vi "test_camera_MAKO.vi"(0 "Boolean 2":bool, 1 "Exposure_set":dbl, 2 "Slide 2":dbl(slide) scale=35.0..1000.0, 3 "Value_Set (ms)":bool, 4 "Bar_Set (ms)":bool, 6 "STOP":bool, 8 "PAUSE":bool, 10 "SAVE PHOTO":bool, 12 "Path":path, 14 "Boolean":bool, 15 "Gain_Set":dbl, 16 "Slide 3":dbl(slide) scale=0.0..30.0, 17 "Bar_Set (dB)":bool, 18 "Value_Set (dB)":bool) -> (5 "gain":dbl, 13 "new picture":picture, 19 "exposure":dbl)   [LabVIEW 2026]
uses:
  <vilib>/picture/picture.llb/Draw True-Color Pixmap.vi
  <userlib>/MakoWrapper/MakoWrapper.lvlib
panel:
  in  "Tab Control 2":enum32{"Image", "Exposure", "Gain"}(tab)
  out "Frame Rate (Hz)":i8
  in  "Duration":dbl
  out "Boolean 3":bool
  out "Frame Flicker":bool
  in  "Start_Video":bool
  in  "Duratin_Video":bool
  out "Auto_Expose":bool
  out "Auto_Gain":bool
  in  "Tab Control":T1(tab)
  out "error_start":errorcluster
  out "start_return":i32
  in  "cameraId":string="DEV_000F315E8832"
  out "error_open":errorcluster
  out "open_return":i32
  out "setup_return":i32
  out "error_setup":errorcluster
  out "error out":errorcluster
  out "error_sizing":errorcluster
  in  "timeoutMs":u32=2000
  in  "bufferSize":u32=4986432
  out "size_return":i32
  out "width":i32
  out "height":i32
  out "outBuffer":u8[](array[numeric])
  out "error_cam_close":errorcluster
  out "cam_close_return":i32
  out "error_shutdown":errorcluster
  out "shutdown_return":i32
  out "error_exposure":errorcluster
  out "exposure_return":i32
  out "error_gain":errorcluster
  out "gain_return":i32
  # "DEV_000F315E8832"
  # "4986432"
  # "2000"
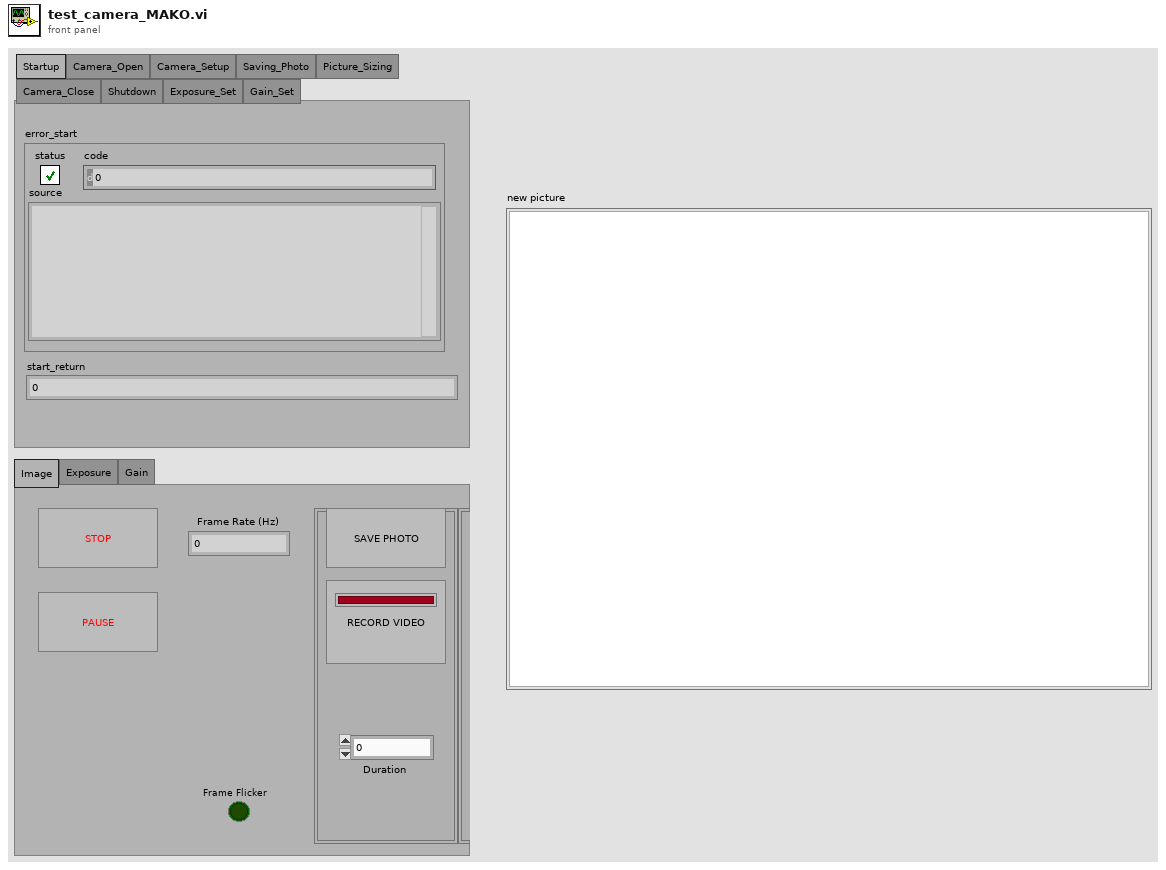
[diagram p1: front panel]
types:
  T1 = enum32{"Startup", "Camera_Open", "Camera_Setup", "Saving_Photo", "Picture_Sizing", "Camera_Close", "Shutdown", "Exposure_Set", "Gain_Set"}
  T2 = typedef "imagedata.ctl" = cluster{"image type":i32, "image depth":i32, "image":u8[], "mask":u8[], "colors":u32[], "Rectangle":cluster{"left":i16, "top":i16, "right":i16, "bottom":i16}}
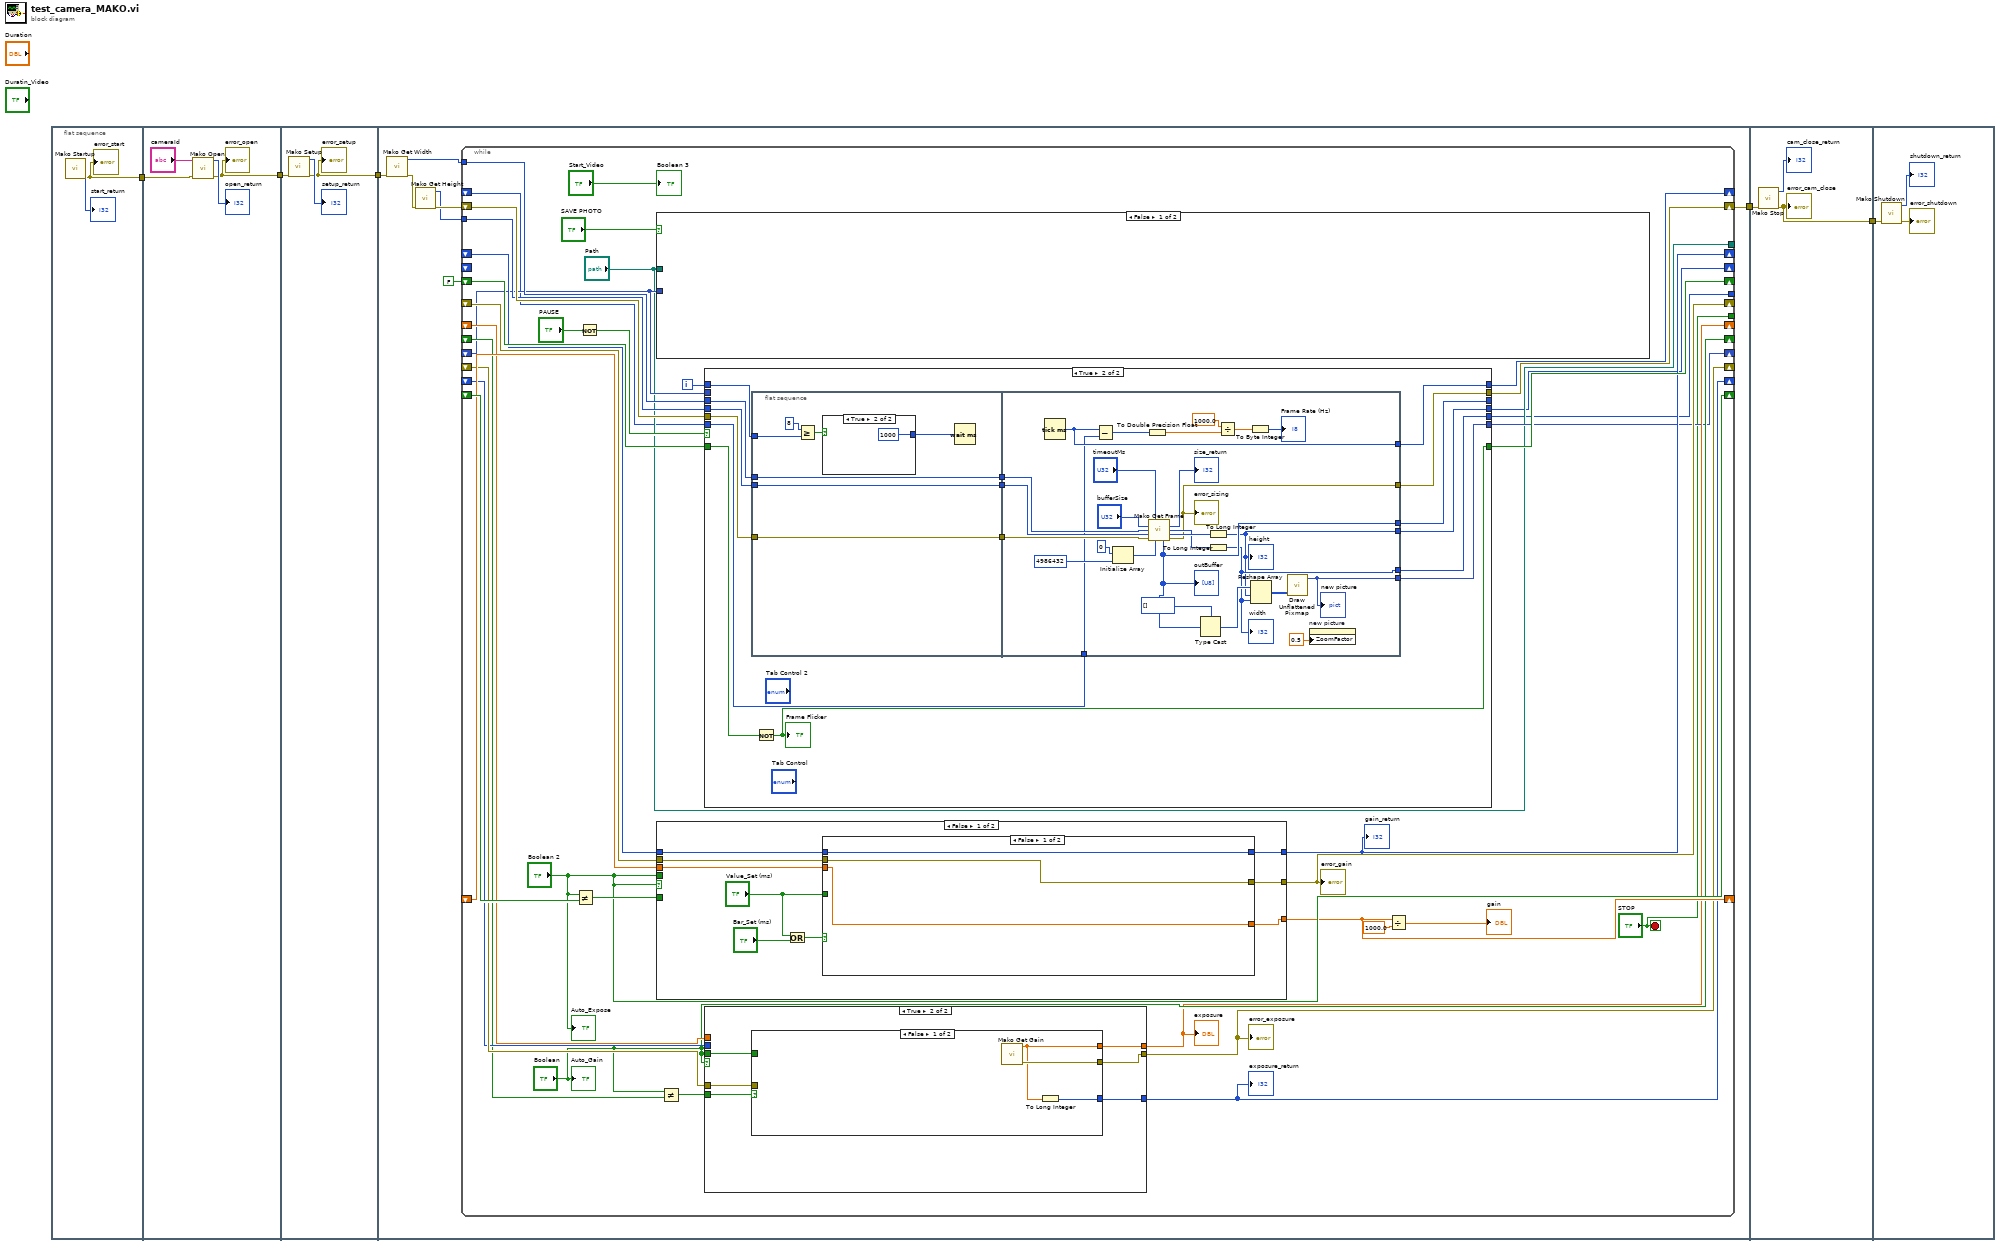
[diagram p0: block diagram]
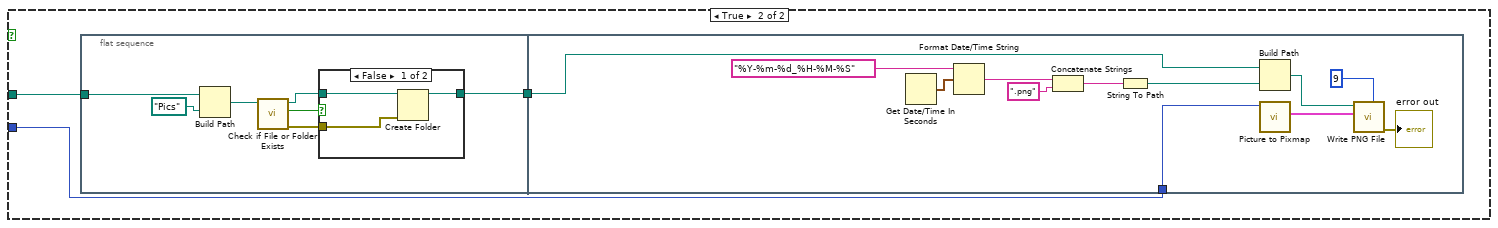
[diagram p2: hidden frame]
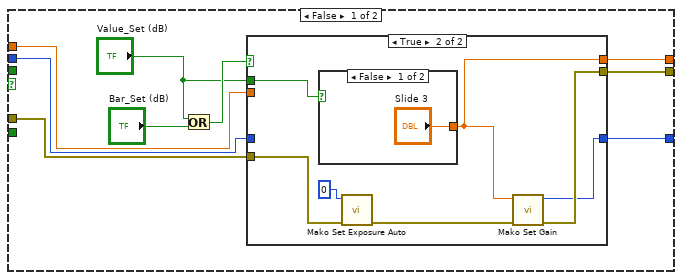
[diagram p4: hidden frame]
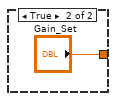
[diagram p6: hidden frame]
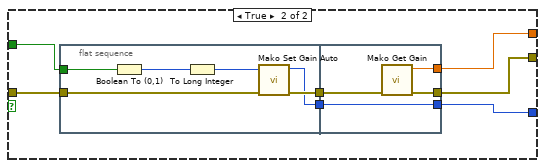
[diagram p7: hidden frame]
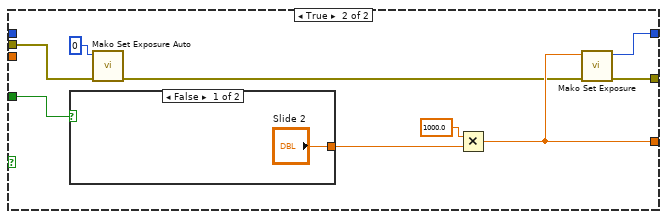
[diagram p8: hidden frame]
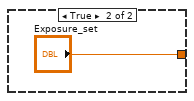
[diagram p9: hidden frame]
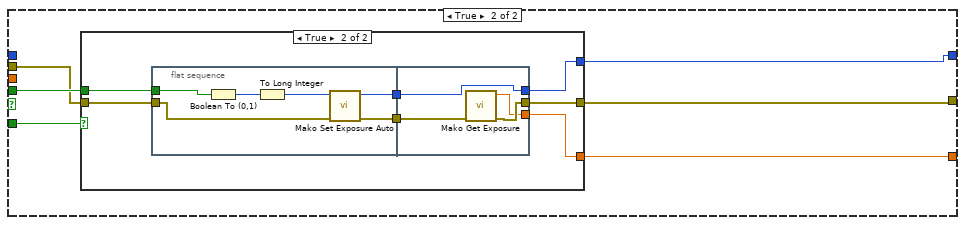
[diagram p10: hidden frame]
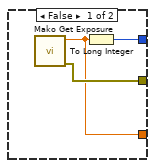
[diagram p11: hidden frame]
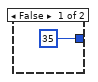
[diagram p13: hidden frame]
diagram:
  n1 = flat-sequence {
    tunnel: [w6] -> w5
    tunnel: w5 -> [w8]
    tunnel: [w9] -> w4
    tunnel: w4 -> [w14]
    tunnel: [w12] -> w3
    tunnel: w3 -> [w21]
    tunnel: [w16] -> w2
    tunnel: w2 -> [w241]
    tunnel: [w239] -> w1
    tunnel: w1 -> [w244]
    frame #0 {
      n2 = call <userlib>:"Mako Startup.vi"() -> ("error out"=w6:errorcluster, "function return"=→"start_return":i32)  [unwired: 10 in]
      "error_start" <- w6
    }
    frame #1 {
      n3 = call <userlib>:"Mako Open.vi"("error in (no error)"=w8, "cameraId"="cameraId") -> ("error out"=w9:errorcluster, "function return"=→"open_return":i32)  [unwired: 8 in]
      "error_open" <- w9
    }
    frame #2 {
      n4 = call <userlib>:"Mako Setup.vi"("error in (no error)"=w14) -> ("error out"=w12:errorcluster, "function return"=→"setup_return":i32)  [unwired: 9 in]
      "error_setup" <- w12
    }
    frame #3 {
      n5 = call <userlib>:"Mako Get Width.vi"("error in (no error)"=w21) -> ("error out"=w20:errorcluster, "function return"=w18:u32)  [unwired: 9 in]
      n6 = call <userlib>:"Mako Get Height.vi"("error in (no error)"=w20) -> ("error out"=w19:errorcluster, "function return"=w17:u32)  [unwired: 9 in]
      n7 = while {
        tunnel: w18 -> [w59]
        tunnel: w17 -> [w58]
        shift-right: [w57] -> w16
        shift-left: w19 -> [w60]
        shift-right: [w52] -> _
        shift-left: FALSE -> [w53]
        shift-right: ["Boolean 2"] -> _
        shift-left: _ -> [w51]
        shift-right: [w48] -> _
        shift-left: _ -> [w47]
        shift-right: [w46] -> _
        shift-left: _ -> [w45]
        shift-right: [w44] -> _
        shift-left: _ -> [w43]
        shift-right: ["Boolean"] -> _
        shift-left: _ -> [w38]
        shift-right: [w36] -> _
        shift-left: _ -> [w40]
        shift-right: [w35] -> _
        shift-left: _ -> [w41]
        shift-right: [w32] -> _
        shift-left: _ -> [w42]
        shift-right: [w30] -> _
        shift-left: _ -> [w29]
        tunnel: ["Path"] -> _
        tunnel: [w26] -> _
        tunnel: ["STOP"] -> _
        shift-right: [w23] -> _
        shift-left: _ -> [w22]
        shift-right: [w25] -> _
        shift-left: _ -> [_]
        i -> [w56]
        stop <- "STOP" stop-if-true
        n8 = Not Equal?(x="Boolean 2", y=w51) -> (x != y?=w50:bool)
        n9 = Not(x="PAUSE") -> (.not. x?=w54:bool)
        n10 = case shown="False" "SAVE PHOTO" {
          tunnel: w29 -> [_ w62]
          tunnel: "Path" -> [_ w61]
          frame False {
          }
          frame True {
            n11 = flat-sequence {
              tunnel: w61 -> [w69]
              tunnel: [w65] -> w63
              tunnel: w63 -> [w84]
              tunnel: w62 -> [w76]
              frame #0 {
                n12 = Build Path(base path=w69, name or relative path=path "Pics") -> (appended path=w64:path)
                n13 = call <vilib>:"Check if File or Folder Exists.vi"("path"=w64) -> ("error out"=w66:errorcluster, "file or folder exists?"=w68:bool, "dup path"=w67:path)  [unwired: 8 in]
                n14 = case shown="False" w68 {
                  tunnel: w67 -> [w73 w74]
                  tunnel: w66 -> [w72 _]
                  tunnel: [w71 w74] -> w65
                  frame False {
                    n15 = Create Folder(path (use dialog)=w73, error in=w72) -> (created path=w71:path)  [unwired: 1 in, 2 out]
                  }
                  frame True {
                  }
                }
              }
              frame #1 {
                n16 = Get Date/Time In Seconds() -> (seconds since 1Jan1904=w86:timestamp)
                n17 = Format Date/Time String(time format string (%c)="%Y-%m-%d_%H-%M-%S", seconds (now)=w86) -> (date/time string=w81:string)  [unwired: 1 in]
                n18 = Concatenate Strings(w81, ".png" ("string")) -> (w82:string)
                n19 = String To Path(string=w82) -> (path=w78:path)
                n20 = Build Path(base path=w84, name or relative path=w78) -> (appended path=w79:path)
                n21 = call <vilib>:"Picture to Pixmap.vi"("picture"=w76) -> ("image data"=w83:T2)  [unwired: 9 in, 1 out]
                n22 = call <vilib>:"Write PNG File.vi"("compression (default)"=9, "image data"=w83, "path to PNG file"=w79) -> ("error out"=→"error out":errorcluster)  [unwired: 7 in, 1 out]
              }
            }
          }
        }
        n23 = case shown="False" "Boolean 2" {
          tunnel: [w139 w158] -> w44
          tunnel: w50 -> [_ w162]
          tunnel: "Boolean 2" -> [_ w161]
          tunnel: [w138 w160] -> w46
          tunnel: [w137 w159] -> w48
          tunnel: w47 -> [w136 _]
          tunnel: w45 -> [w135 w157]
          tunnel: w43 -> [w134 _]
          frame False {
            n24 = Or(x="Value_Set (ms)", y="Bar_Set (ms)") -> (x .or. y?=w142:bool)
            n25 = case shown="False" w142 {
              tunnel: [w143 w150] -> w139
              tunnel: "Value_Set (ms)" -> [_ w154]
              tunnel: [w144 w153] -> w138
              tunnel: [w145 w152] -> w137
              tunnel: w136 -> [w145 _]
              tunnel: w135 -> [w144 w148]
              tunnel: w134 -> [w143 _]
              frame False {
              }
              frame True {
                n26 = case shown="False" w154 {
                  tunnel: ["Slide 2" "Exposure_set"] -> w151
                  frame False {
                  }
                  frame True {
                  }
                }
                n27 = call <userlib>:"Mako Set Exposure Auto.vi"("error in (no error)"=w148, "autoOn"=0) -> ("error out"=w147:errorcluster)  [unwired: 8 in, 1 out]
                n28 = Multiply(x=1000.0, y=w151) -> (x*y=w150:dbl)
                n29 = call <userlib>:"Mako Set Exposure.vi"("error in (no error)"=w147, "exposureUs"=w150) -> ("error out"=w153:errorcluster, "function return"=w152:i32)  [unwired: 8 in]
              }
            }
          }
          frame True {
            n30 = case shown="True" w162 {
              tunnel: w161 -> [_ w172]
              tunnel: [w165 w171] -> w160
              tunnel: [w164 w170] -> w159
              tunnel: [w163 w167] -> w158
              tunnel: w157 -> [_ w166]
              frame False {
                n31 = call <userlib>:"Mako Get Exposure.vi"() -> ("error out"=w165:errorcluster, "function return"=w163:dbl)  [unwired: 10 in]
                n32 = To Long Integer(number=w163) -> (32bit integer=w164:i32)
              }
              frame True {
                n33 = flat-sequence {
                  tunnel: w172 -> [w178]
                  tunnel: [w175] -> w169
                  tunnel: [w174] -> w168
                  tunnel: w166 -> [w173]
                  tunnel: [w182] -> w170
                  tunnel: [w180] -> w171
                  tunnel: w169 -> [w181]
                  tunnel: w168 -> [w182]
                  tunnel: [w179] -> w167
                  frame #0 {
                    n34 = Boolean To (0,1)(Boolean=w178) -> (0, 1=w177:i16)
                    n35 = To Long Integer(number=w177) -> (32bit integer=w176:i32)
                    n36 = call <userlib>:"Mako Set Exposure Auto.vi"("error in (no error)"=w173, "autoOn"=w176) -> ("error out"=w175:errorcluster, "function return"=w174:i32)  [unwired: 8 in]
                  }
                  frame #1 {
                    n37 = call <userlib>:"Mako Get Exposure.vi"("error in (no error)"=w181) -> ("error out"=w180:errorcluster, "function return"=w179:dbl)  [unwired: 9 in]
                  }
                }
              }
            }
          }
        }
        "error_gain" <- w46
        "gain_return" <- w48
        n38 = Not Equal?(x="Boolean", y=w38) -> (x != y?=w39:bool)
        n39 = case shown="True" w54 {
          tunnel: w60 -> [w186 w202]
          tunnel: w59 -> [_ w197]
          tunnel: w58 -> [_ w201]
          tunnel: [w186 w200] -> w57
          tunnel: w56 -> [_ w193]
          tunnel: w53 -> [w185 w199]
          tunnel: [w185 w198] -> w52
          tunnel: [w184 w192] -> w30
          tunnel: w29 -> [w184 _]
          tunnel: [_ w191] -> _
          tunnel: [_ w190] -> w26
          tunnel: [_ w189] -> w25
          tunnel: [w183 w188] -> w23
          tunnel: w22 -> [w183 w187]
          frame False {
          }
          frame True {
            n40 = flat-sequence {
              tunnel: w197 -> [w207]
              tunnel: w201 -> [w208]
              tunnel: w202 -> [w209]
              tunnel: [w209] -> w196
              tunnel: [w208] -> w195
              tunnel: [w207] -> w194
              tunnel: w193 -> [w203]
              tunnel: w196 -> [w238]
              tunnel: w195 -> [w226]
              tunnel: w194 -> [w225]
              tunnel: [w231] -> w200
              tunnel: [w223] -> w192
              tunnel: [w222] -> w191
              tunnel: [w221] -> w190
              tunnel: [w220] -> w189
              tunnel: [w218] -> w188
              tunnel: w187 -> [w217]
              frame #0 {
                n41 = Greater Or Equal?(x=8, y=w203) -> (x >= y?=w205:bool)
                n42 = case shown="True" w205 {
                  tunnel: [u32 35 ("milliseconds to wait") u32 1000 ("milliseconds to wait")] -> w204
                  frame False {
                  }
                  frame True {
                  }
                }
                n43 = Wait (ms)(milliseconds to wait=w204) -> ()  [unwired: 1 out]
              }
              frame #1 {
                n44 = Tick Count (ms)() -> (millisecond timer value=w218:u32)
                n45 = Subtract(x=w218, y=w217) -> (x-y=w219:u32)
                n46 = Initialize Array(u8 0 ("element"), 4986432 ("dimension size")) -> (w228:u8[])
                n47 = To Double Precision Float(number=w219) -> (double precision float=w214:dbl)
                n48 = call <userlib>:"Mako Get Frame.vi"("timeoutMs"="timeoutMs", "bufferSize"="bufferSize", "outWidth"=w225, "outHeight"=w226, "error in (no error)"=w238, "outBuffer"=w228) -> ("function return"=→"size_return":i32, "outWidth out"=w232:u32, "outHeight out"=w233:u32, "outBuffer 2"=w222:u8[], "error out"=w231:errorcluster)  [unwired: 5 in]
                "error_sizing" <- w231
                "outBuffer" <- w222
                n49 = Type Cast(type=u32[] [] ("data (RGB format)"), x=w222) -> (*(type *) &x=w235:u32[])
                n50 = To Long Integer(number=w233) -> (32bit integer=w220:i32)
                "height" <- w220
                n51 = To Long Integer(number=w232) -> (32bit integer=w221:i32)
                "width" <- w221
                n52 = Divide(x=1000.0, y=w214) -> (x/y=w216:dbl)
                n53 = To Byte Integer(number=w216) -> (8bit integer=→"Frame Rate (Hz)":i8)
                n54 = Reshape Array(w235, w220, w221) -> (w224:u32[][])
                n55 = call-poly <vilib>:"Draw Unflattened Pixmap.vi"("data (RGB format)"=w224) -> ("new picture"=w223:picture)  [unwired: 8 in]
                "new picture" <- w223
                n56 = property on="new picture" class="Pict"("ZoomFactor"=sgl 0.5 ("Zoom Factor")) -> ()  [unwired: 2 in, 2 out]
              }
            }
            n57 = Not(x=w199) -> (.not. x?=w198:bool)
            "Frame Flicker" <- w198
          }
        }
        n58 = case shown="True" "Boolean" {
          tunnel: [w94 w109] -> w32
          tunnel: w39 -> [_ w113]
          tunnel: "Boolean" -> [_ w112]
          tunnel: [w93 w111] -> w35
          tunnel: [w92 w110] -> w36
          tunnel: w40 -> [w91 _]
          tunnel: w41 -> [w90 w108]
          tunnel: w42 -> [w89 _]
          frame False {
            n59 = Or(x="Value_Set (dB)", y="Bar_Set (dB)") -> (x .or. y?=w95:bool)
            n60 = case shown="True" w95 {
              tunnel: [w96 w102] -> w94
              tunnel: "Value_Set (dB)" -> [_ w105]
              tunnel: [w97 w104] -> w93
              tunnel: [w98 w103] -> w92
              tunnel: w91 -> [w98 _]
              tunnel: w90 -> [w97 w100]
              tunnel: w89 -> [w96 _]
              frame False {
              }
              frame True {
                n61 = case shown="False" w105 {
                  tunnel: ["Slide 3" "Gain_Set"] -> w102
                  frame False {
                  }
                  frame True {
                  }
                }
                n62 = call <userlib>:"Mako Set Exposure Auto.vi"("error in (no error)"=w100, "autoOn"=0) -> ("error out"=w99:errorcluster)  [unwired: 8 in, 1 out]
                n63 = call <userlib>:"Mako Set Gain.vi"("error in (no error)"=w99, "gain"=w102) -> ("error out"=w104:errorcluster, "function return"=w103:i32)  [unwired: 8 in]
              }
            }
          }
          frame True {
            n64 = case shown="False" w113 {
              tunnel: w112 -> [_ w123]
              tunnel: [w116 w122] -> w111
              tunnel: [w115 w121] -> w110
              tunnel: [w114 w118] -> w109
              tunnel: w108 -> [_ w117]
              frame False {
                n65 = call <userlib>:"Mako Get Gain.vi"() -> ("error out"=w116:errorcluster, "function return"=w114:dbl)  [unwired: 10 in]
                n66 = To Long Integer(number=w114) -> (32bit integer=w115:i32)
              }
              frame True {
                n67 = flat-sequence {
                  tunnel: w123 -> [w129]
                  tunnel: [w126] -> w120
                  tunnel: [w125] -> w119
                  tunnel: w117 -> [w124]
                  tunnel: [w133] -> w121
                  tunnel: [w131] -> w122
                  tunnel: w120 -> [w132]
                  tunnel: w119 -> [w133]
                  tunnel: [w130] -> w118
                  frame #0 {
                    n68 = Boolean To (0,1)(Boolean=w129) -> (0, 1=w128:i16)
                    n69 = To Long Integer(number=w128) -> (32bit integer=w127:i32)
                    n70 = call <userlib>:"Mako Set Gain Auto.vi"("error in (no error)"=w124, "autoOn"=w127) -> ("error out"=w126:errorcluster, "function return"=w125:i32)  [unwired: 8 in]
                  }
                  frame #1 {
                    n71 = call <userlib>:"Mako Get Gain.vi"("error in (no error)"=w132) -> ("error out"=w131:errorcluster, "function return"=w130:dbl)  [unwired: 9 in]
                  }
                }
              }
            }
          }
        }
        "exposure" <- w32
        "exposure_return" <- w36
        "error_exposure" <- w35
        n72 = Divide(x=w44, y=1000.0) -> (x/y=→"gain":dbl)
        "Auto_Expose" <- "Boolean 2"
        "Auto_Gain" <- "Boolean"
        "Boolean 3" <- "Start_Video"
      }
    }
    frame #4 {
      n73 = call <userlib>:"Mako Stop.vi"("error in (no error)"=w241) -> ("error out"=w239:errorcluster, "function return"=→"cam_close_return":i32)  [unwired: 9 in]
      "error_cam_close" <- w239
    }
    frame #5 {
      n74 = call <userlib>:"Mako Shutdown.vi"("error in (no error)"=w244) -> ("error out"=→"error_shutdown":errorcluster, "function return"=→"shutdown_return":i32)  [unwired: 9 in]
    }
  }
